vi "Initialize.vi"(8 "error in (no error)":errorcluster, 11 "BufferTest in":refnum<class "BufferTest.lvclass">) -> (0 "error out":errorcluster, 3 "BufferTest out":refnum<class "BufferTest.lvclass">)   [LabVIEW 2017, in "DSFPluginTest.lvlib" / "BufferTest.lvclass"]
uses:
  BufferTest.lvclass
  builds/Data Sharing Framework/Current/Data Sharing Framework Core/DSF Core.lvlibp/Engine/Classes/Buffer Converter/Buffer Converter.lvclass
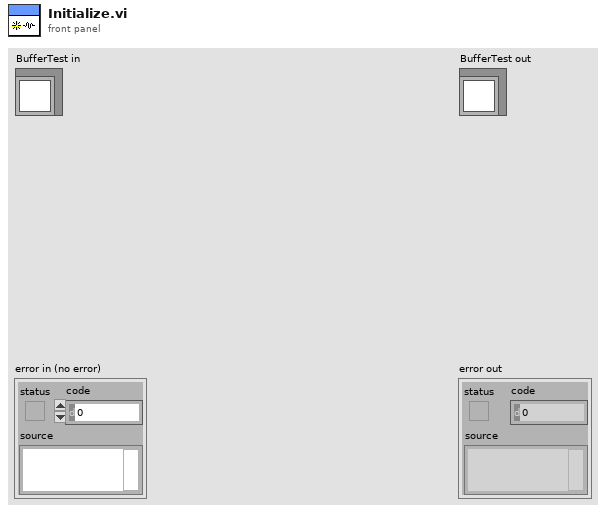
[diagram p1: front panel]
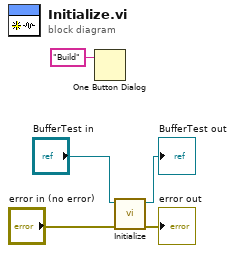
[diagram p0: block diagram]
diagram:
  n1 = One Button Dialog(message="Build") -> ()  [unwired: 1 in, 1 out]
  n2 = call-parent "Initialize.vi"("error in (no error)"="error in (no error)", "Buffer Converter in"="BufferTest in") -> ("error out"=→"error out":errorcluster, "Buffer Converter out"=→"BufferTest out":refnum<class "BufferTest.lvclass">)  [unwired: 8 in]
